vi "SS Configure 1.vi"(4 "Flow Control":T1, 6 "Parity":T2, 7 "Stop Bits":T3, 8 "error in (no error)":errorcluster, 9 "Data Bits":T4=enum."8", 10 "Baud Rate":T5=enum."9600 bps", 11 "Simple Serial Ref in":T6) -> (0 "error out":errorcluster, 3 "Simple Serial Ref out":T6)   [LabVIEW 2009]
uses:
  SS FPGA VI Ref.ctl
  <vilib>/LabVIEW Targets/FPGA/cRIO/shared/nicrio_ModuleControls/nicrio_cRIO-9871_BaudRateEnum.ctl
  <vilib>/LabVIEW Targets/FPGA/cRIO/shared/nicrio_ModuleControls/nicrio_cRIO-9871_DataBitsEnum.ctl
  <vilib>/LabVIEW Targets/FPGA/cRIO/shared/nicrio_ModuleControls/nicrio_cRIO-9871_StopBitsEnum.ctl
  <vilib>/LabVIEW Targets/FPGA/cRIO/shared/nicrio_ModuleControls/nicrio_cRIO-9871_ParityEnum.ctl
  <vilib>/LabVIEW Targets/FPGA/cRIO/shared/nicrio_ModuleControls/nicrio_cRIO-9871_FlowControlEnum.ctl
  <vilib>/rvi/interface/nirviReadWriteControl/nirviReadWriteControl.xnode
  FPGA Bitfiles/Q_IGVC_2010.lvproj_FPGA Target_GPS diagnostic.vi.lvbitx
  <vilib>/Utility/error.llb/Error Cluster From Error Code.vi
  <vilib>/rvi/errors/niLvFpgaAdjustHostInterfaceError.vi
  <vilib>/rvi/interface/common/niFpgaNodeNameForErrorReporting.ctl
  <vilib>/rvi/errors/niLvFpgaWhatHappensToTopLevelVI.ctl
  <vilib>/rvi/interface/nirviMethod/nirviMethod.xnode
  <vilib>/LabVIEW Targets/FPGA/RIO/nirio_HostInterface/nirio_WaitOnIRQ.vi
  <vilib>/RVI Host/nirviSupport.llb/nirviErrorClusterFromErrorCode.vi
  NiRioSrv.dll
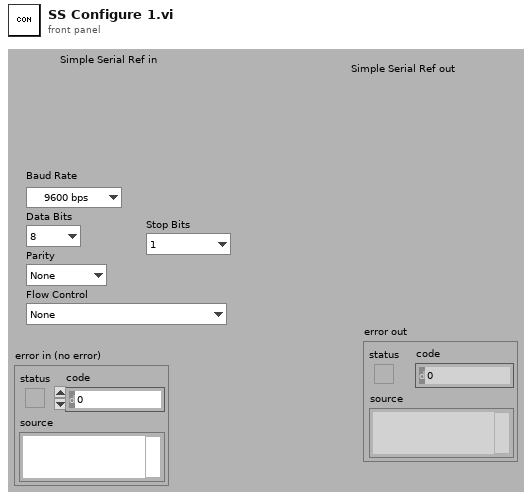
[diagram p1: front panel]
types:
  T1 = typedef "nicrio_cRIO-9871_FlowControlEnum.ctl" = enum8{"None", "Software (XON / XOFF)", "Hardware (RTS / CTS)"}
  T2 = typedef "nicrio_cRIO-9871_ParityEnum.ctl" = enum8{"None", "Odd", "Even", "Mark", "Space"}
  T3 = typedef "nicrio_cRIO-9871_StopBitsEnum.ctl" = enum8{"1", "1.5", "2"}
  T4 = typedef "nicrio_cRIO-9871_DataBitsEnum.ctl" = enum8{"5", "6", "7", "8"}
  T5 = typedef "nicrio_cRIO-9871_BaudRateEnum.ctl" = enum16{"75 bps", "110 bps", "134 bps", "150 bps", "300 bps", "600 bps", "1200 bps", "1800 bps", "2400 bps", "4800 bps", "7200 bps", "9600 bps", "14.4 kbps", "19.2 kbps", "28.8 kbps", "38.4 kbps", "57.6 kbps", "115.2 kbps", "230.4 kbps", "460.8 kbps", "921.6 kbps"}
  T6 = typedef "SS FPGA VI Ref.ctl" = refnum<k20>
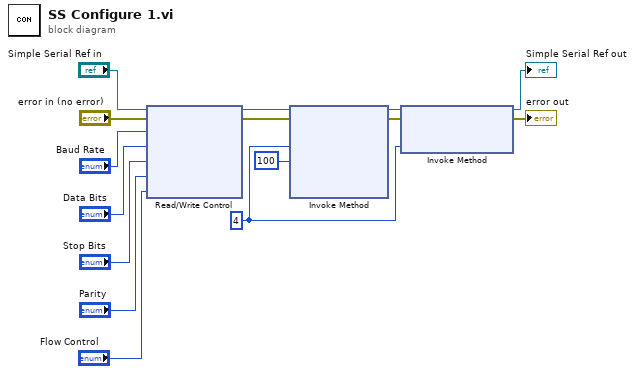
[diagram p0: block diagram]
diagram:
  w5 = 4 ("Port 1 wait for start IRQ")
  n1 = xnode "Read/Write Control"("FPGA VI Reference In"="Simple Serial Ref in", "error in"="error in (no error)", "Baud Rate 1"="Baud Rate", "Data Bits 1"="Data Bits", "Stop Bits 1"="Stop Bits", "Parity 1"="Parity", "Flow Control 1"="Flow Control") -> ("FPGA VI Reference Out"=w7:T6, "error out"=w6:errorcluster)
  n2 = xnode "Invoke Method"("FPGA VI Reference In"=w7, "error in"=w6, "IRQ Number(s)"=w5, "Timeout (ms)"=100) -> ("FPGA VI Reference Out"=w9:T6, "error out"=w8:errorcluster)  [unwired: 2 out]
  n3 = xnode "Invoke Method"("FPGA VI Reference In"=w9, "error in"=w8, "IRQ Number(s)"=w5) -> ("FPGA VI Reference Out"=→"Simple Serial Ref out":T6, "error out"=→"error out":errorcluster)
